vi "SeCrTS-DD Log Analog Queues.vi"(8 "error in":errorcluster, 9 "Analog queues":refnum<queue>[](array[refnum]), 10 "Channel names":T1, 11 "tdms file in":refnum<k34>) -> (0 "error out":errorcluster, 3 "tdms ref out":refnum<k34>)   [LabVIEW 2022 SP3]
uses:
  <vilib>/Waveform/WDTOps.llb/WDT Get Waveform Time Array DBL.vi
panel:
  out "x":u32
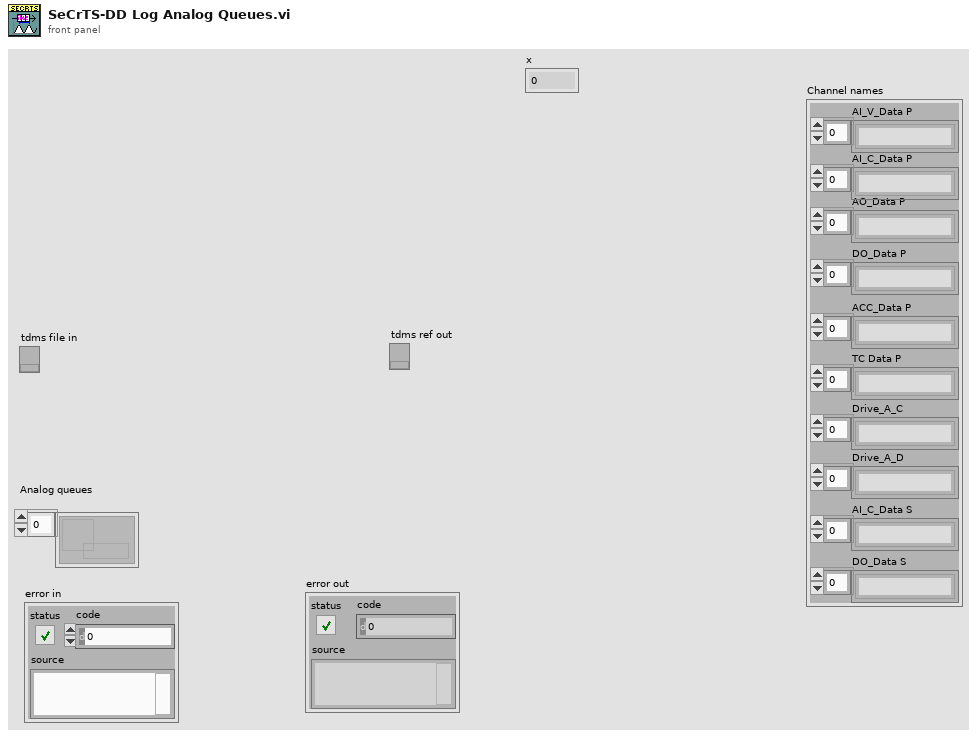
[diagram p1: front panel]
types:
  T1 = cluster{"AI_C_Data P":string[], "AI_V_Data P":string[], "AO_Data P":string[], "DO_Data P":string[], "ACC_Data P":string[], "TC Data P":string[], "Drive_A_C":string[], "Drive_A_D":string[], "AI_C_Data S":string[], "DO_Data S":string[]}
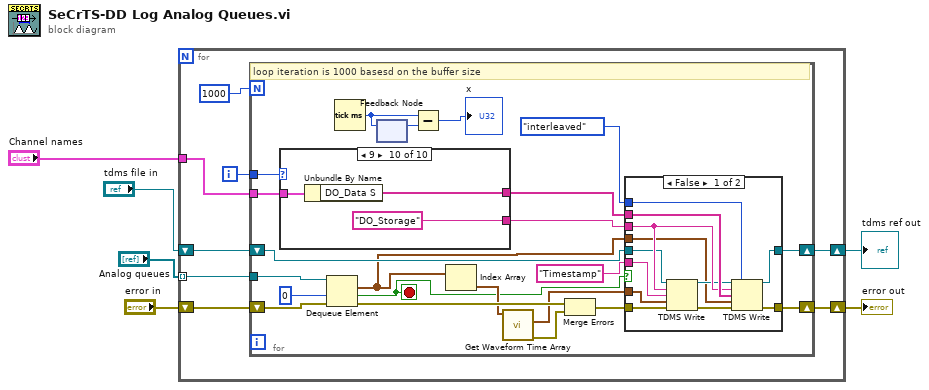
[diagram p0: block diagram]
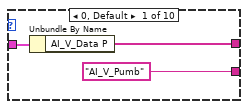
[diagram p3: hidden frame]
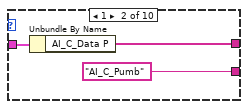
[diagram p4: hidden frame]
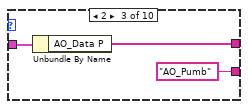
[diagram p5: hidden frame]
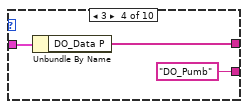
[diagram p6: hidden frame]
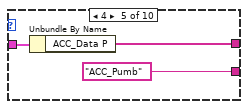
[diagram p7: hidden frame]
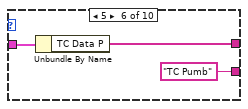
[diagram p8: hidden frame]
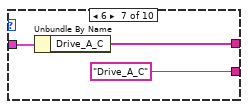
[diagram p9: hidden frame]
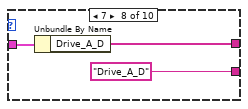
[diagram p10: hidden frame]
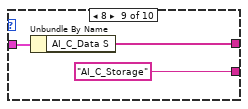
[diagram p11: hidden frame]
diagram:
  n1 = for {
    tunnel: "Analog queues" -> [w13] mode=indexing
    shift-right: [w11] -> w4
    shift-left: "tdms file in" -> [w14]
    shift-right: [w9] -> w3
    shift-left: "error in" -> [w10]
    tunnel: "Channel names" -> [w7]
    i -> [w8]
    n2 = for {
      N: 1000 -> [_]
      tunnel: w13 -> [w32]
      shift-right: [w22] -> w11
      shift-left: w14 -> [w23]
      shift-right: [w28] -> w9
      shift-left: w10 -> [w31]
      tunnel: w8 -> [w36]
      tunnel: w7 -> [w20]
      stop <- w19 stop-if-true
      # "loop iteration is 1000 basesd on the buffer size"
      n3 = case shown="9" w36 {
        tunnel: [w51 w54 w57 w60 w63 w66 w69 w72 w75 w78] -> w27
        tunnel: ["AI_V_Pumb" ("group name in (Untitled)") "AI_C_Pumb" ("group name in (Untitled)") "AO_Pumb" ("group name in (Untitled)") "DO_Pumb" ("group name in (Untitled)") "ACC_Pumb" ("group name in (Untitled)") "TC Pumb" ("group name in (Untitled)") "Drive_A_C" ("group name in (Untitled)") "Drive_A_D" ("group name in (Untitled)") "AI_C_Storage" ("group name in (Untitled)") "DO_Storage" ("group name in (Untitled)")] -> w26
        tunnel: w20 -> [w52 w55 w58 w61 w64 w67 w70 w73 w76 w79]
        frame 0, Default {
          n4 = Unbundle By Name(w52) -> ("AI_V_Data P"=w51:string[])
        }
        frame 1 {
          n5 = Unbundle By Name(w55) -> ("AI_C_Data P"=w54:string[])
        }
        frame 2 {
          n6 = Unbundle By Name(w58) -> ("AO_Data P"=w57:string[])
        }
        frame 3 {
          n7 = Unbundle By Name(w61) -> ("DO_Data P"=w60:string[])
        }
        frame 4 {
          n8 = Unbundle By Name(w64) -> ("ACC_Data P"=w63:string[])
        }
        frame 5 {
          n9 = Unbundle By Name(w67) -> ("TC Data P"=w66:string[])
        }
        frame 6 {
          n10 = Unbundle By Name(w70) -> ("Drive_A_C"=w69:string[])
        }
        frame 7 {
          n11 = Unbundle By Name(w73) -> ("Drive_A_D"=w72:string[])
        }
        frame 8 {
          n12 = Unbundle By Name(w76) -> ("AI_C_Data S"=w75:string[])
        }
        frame 9 {
          n13 = Unbundle By Name(w79) -> ("DO_Data S"=w78:string[])
        }
      }
      n14 = Dequeue Element(queue=w32, timeout in ms (-1)=0, error in (no error)=w31) -> (element=w18:waveform(dbl)[], timed out?=w19:bool, error out=w34:errorcluster)  [unwired: 1 out]
      n15 = Tick Count (ms)() -> (millisecond timer value=w16:u32)
      n16 = feedback #1() -> (w17:u32)  [unwired: 1 in]
      n17 = feedback-in #1(w16) -> ()
      n18 = Subtract(x=w16, y=w17) -> (x-y=→"x":u32)
      n19 = Index Array(array=w18) -> (element=w30:waveform(dbl))  [unwired: 1 in]
      n20 = call-poly <vilib>:"Get Waveform Time Array.vi"("waveform in"=w30) -> ("error out"=w33:errorcluster, "X array"=w24:timestamp[])  [unwired: 9 in]
      n21 = Merge Errors(w34, w33) -> (w29:errorcluster)
      n22 = case shown="False" w19 {
        tunnel: w29 -> [w48 w50]
        tunnel: [w46 w50] -> w28
        tunnel: w27 -> [w45 _]
        tunnel: w26 -> [w44 _]
        tunnel: "Timestamp" -> [w43 _]
        tunnel: w24 -> [w42 _]
        tunnel: w23 -> [w41 w49]
        tunnel: [w39 w49] -> w22
        tunnel: w18 -> [w38 _]
        tunnel: enum16{"decimated", "interleaved"}."interleaved" ("data layout (0:decimated)") -> [w37 _]
        frame False {
          n23 = TDMS Write(0:w41, 5:w44, 7:w43, 9:w42, 11:w48) -> (4:w40:refnum<k34>, 15:w47:errorcluster)  [unwired: 1 in, 2 out]
          n24 = TDMS Write(0:w40, 1:w37, 5:w44, 7:w45, 9:w38, 11:w47) -> (4:w39:refnum<k34>, 15:w46:errorcluster)  [unwired: 2 out]
        }
        frame True {
        }
      }
    }
  }
  "tdms ref out" <- w4
  "error out" <- w3
